vi "CreateClassColored.vi"() -> ()   [LabVIEW 2014]
panel:
  in  "Wire Pens":T1(array[cluster])=[{"Foreground Color"=0, "Background Color"=0, "Fill Pattern"={"Row 0"=0, "Row 1"=0, "Row 2"=0, "Row 3"=0, "Row 4"=0, "Row 5"=0, "Row 6"=0, "Row 7"=0}, "Width"=0, "Mode"=enum."Copy", "Style"=enum."Solid", "Fill Rule"=enum."Even Odd", "End Caps"=enum."Default"}, {"Foreground Color"=4294967295, "Background Color"=4294967295, "Fill Pattern"={"Row 0"=0, "Row 1"=0, "Row 2"=0, "Row 3"=0, "Row 4"=0, "Row 5"=0, "Row 6"=0, "Row 7"=0}, "Width"=3, "Mode"=enum."Copy", "Style"=enum."Solid", "Fill Rule"=enum."Even Odd", "End Caps"=enum."Default"}]
  out "x+1":i32
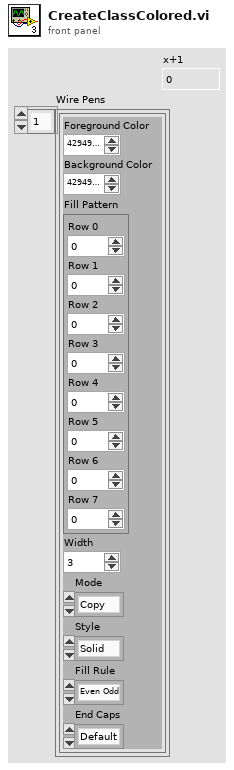
[diagram p1: front panel]
types:
  T1 = cluster{"Foreground Color":u32, "Background Color":u32, "Fill Pattern":cluster{"Row 0":u8, "Row 1":u8, "Row 2":u8, "Row 3":u8, "Row 4":u8, "Row 5":u8, "Row 6":u8, "Row 7":u8}, "Width":i16, "Mode":enum16{"Copy", "Or", "Exclusive Or", "Bit Clear", "Not Copy", "Not Or", "Nor Exclusive Or", "Not Bit Clear"}, "Style":enum32{"Solid", "Dash", "Dot", "Dash Dot", "Dash Dot Dot"}, "Fill Rule":enum32{"Even Odd", "Winding"}, "End Caps":enum32{"Default", "Flat"}}[]
  T2 = cluster{"Foreground Color":u32, "Background Color":u32, "Fill Pattern":cluster{"Row 0":u8, "Row 1":u8, "Row 2":u8, "Row 3":u8, "Row 4":u8, "Row 5":u8, "Row 6":u8, "Row 7":u8}, "Width":i16, "Mode":enum16{"Copy", "Or", "Exclusive Or", "Bit Clear", "Not Copy", "Not Or", "Nor Exclusive Or", "Not Bit Clear"}, "Style":enum32{"Solid", "Dash", "Dot", "Dash Dot", "Dash Dot Dot"}, "Fill Rule":enum32{"Even Odd", "Winding"}, "End Caps":enum32{"Default", "Flat"}}
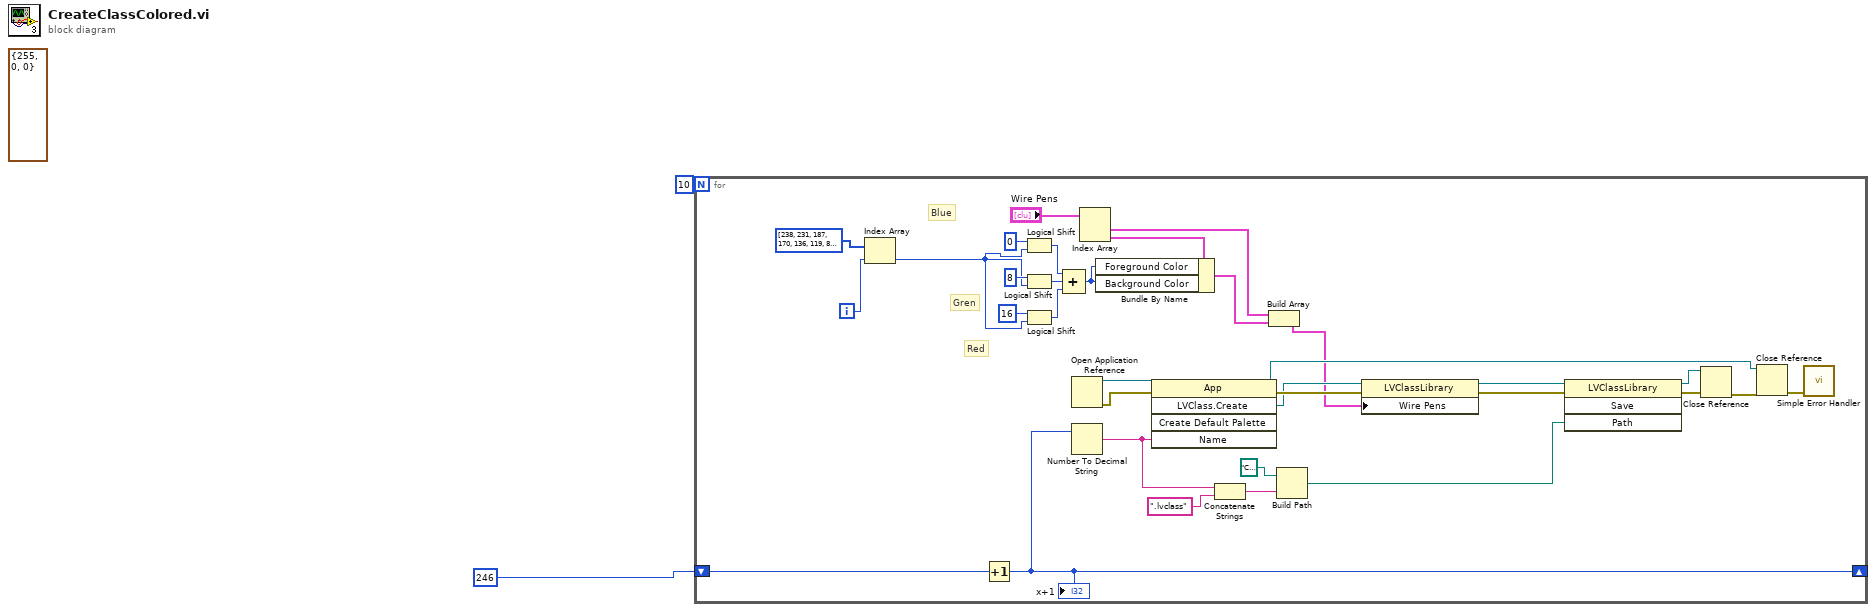
[diagram p0: block diagram]
diagram:
  (unwired) cluster{"Blue":u32, "Green":u32, "Red":u32} {"Blue"=255, "Green"=0, "Red"=0}
  n1 = for {
    N: 10 -> [_]
    shift-right: [w6] -> _
    shift-left: 246 -> [w7]
    i -> [w4]
    # "Red"
    # "Gren"
    # "Blue"
    n2 = Index Array(array=u32[] [238, 231, 187, 170, 136, 119, 86, 68, 34, 17], index=w4) -> (element=w3:u32)
    n3 = Increment(x=w7) -> (x+1=w6:i32)
    "x+1" <- w6
    n4 = Logical Shift(y=i16 0, x=w3) -> (x << y=w14:u32)
    n5 = Logical Shift(y=i16 8, x=w3) -> (x << y=w13:u32)
    n6 = Logical Shift(y=i16 16, x=w3) -> (x << y=w12:u32)
    n7 = Compound Arithmetic op=ADD(w14, w13, w12) -> (w8:u32)
    n8 = Open Application Reference() -> (0:w34:errorcluster, 3:w35:refnum<vi>)  [unwired: 4 in]
    n9 = Number To Decimal String(number=w6) -> (decimal integer string=w15:string)  [unwired: 1 in]
    n10 = Index Array(array="Wire Pens") -> (element #1=w17:T2, element #2=w19:T2)  [unwired: 2 in]
    n11 = Bundle By Name(cluster=w19, "Foreground Color"=w8, "Background Color"=w8) -> (w18:T2)
    n12 = invoke class="App" method="LVClass.Create"(reference=w35, error in=w34, "Name"=w15) -> (reference out=w25:refnum<vi>, error out=w33:errorcluster, "LVClass.Create"=w22:refnum<vi>)  [unwired: 2 in, 2 out]
    n13 = Concatenate Strings(w15, ".lvclass") -> (w31:string)
    n14 = Build Array(w17, w18) -> (w16:T1)
    n15 = Build Path(base path=path "C:/Users/mjacobso/Desktop/Create Color/Colors", name or relative path=w31) -> (appended path=w29:path)
    n16 = property class="LVClassLibrary"(reference=w22, error in=w33, "Wire Pens"=w16) -> (reference out=w21:refnum<vi>, error out=w23:errorcluster)
    n17 = invoke class="LVClassLibrary" method="Save"(reference=w21, error in=w23, "Path"=w29) -> (reference out=w26:refnum<vi>, error out=w27:errorcluster)  [unwired: 1 in, 2 out]
    n18 = Close Reference(reference=w26, error in (no error)=w27) -> (error out=w28:errorcluster)
    n19 = Close Reference(reference=w25, error in (no error)=w28) -> (error out=w24:errorcluster)
    n20 = call <vilib>:"Simple Error Handler.vi"("error in (no error)"=w24) -> ()  [unwired: 4 in, 5 out]
  }
